vi "ReadWriteLoopCase1.vi"() -> ()   [LabVIEW 2019]
uses:
  <vilib>/DAQmx/read.llb/DAQmx Read (Analog DBL 1Chan 1Samp).vi
  <vilib>/DAQmx/write.llb/DAQmx Write (Analog DBL 1Chan 1Samp).vi
  <vilib>/DAQmx/create/channels.llb/DAQmx Create Channel (AI-Voltage-Basic).vi
  <vilib>/DAQmx/configure/timing.llb/DAQmx Timing (Sample Clock).vi
  <vilib>/DAQmx/create/channels.llb/DAQmx Create Channel (AO-Voltage-Basic).vi
  <vilib>/DAQmx/miscellaneous.llb/DAQmx Fill In Error Info.vi
panel:
  out "error out":errorcluster
  out "Slide":dbl(slide) scale=2900.0..3100.0
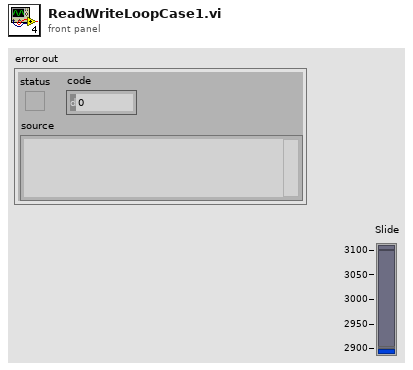
[diagram p1: front panel]
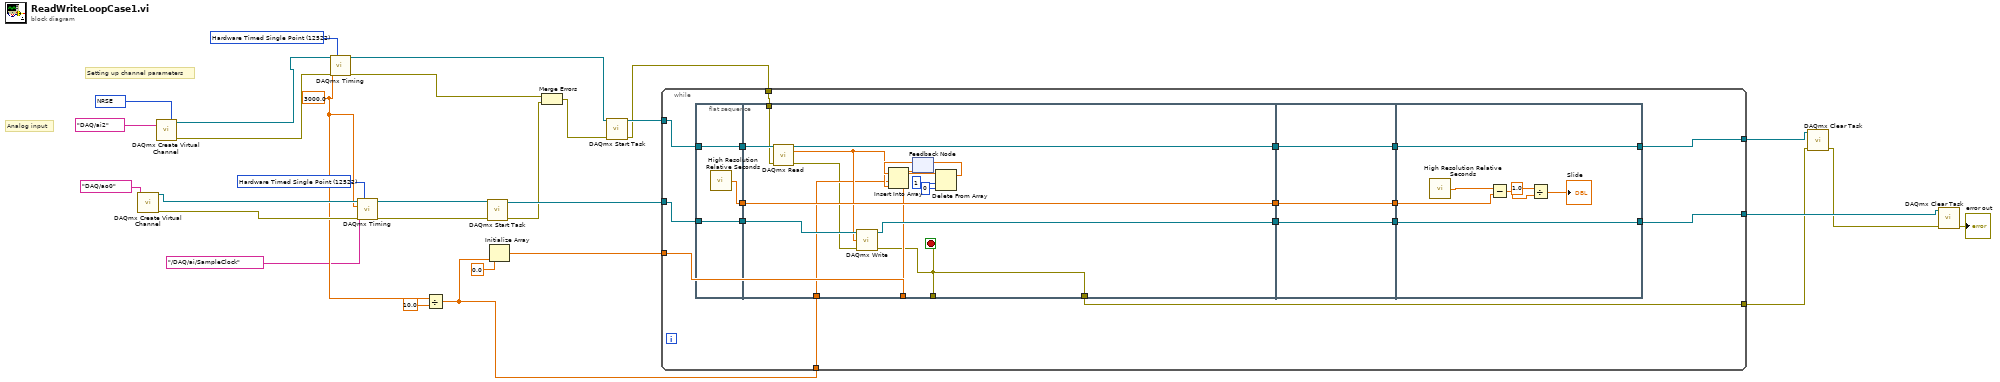
[diagram p0: block diagram]
diagram:
  w3 = 12522 items=["Finite Samples"=10178, "Continuous Samples"=10123, "Hardware Timed Single Point"=12522] ("sample mode")
  w4 = 3000.0 ("rate")
  w24 = 12522 items=["Finite Samples"=10178, "Continuous Samples"=10123, "Hardware Timed Single Point"=12522] ("sample mode")
  w27 = 10078 items=["Default"=-1, "RSE"=10083, "NRSE"=10078, "Differential"=10106, "Pseudodifferential"=12529] ("input terminal configuration")
  # "Analog input"
  # "Setting up channel parameters"
  n1 = call-poly <vilib>:"DAQmx Create Virtual Channel.vi"("physical channels"=tag "DAQ/ao0") -> ("task out"=w8:refnum<k21>, "error out"=w6:errorcluster)  [unwired: 13 in]
  n2 = call-poly <vilib>:"DAQmx Create Virtual Channel.vi"("input terminal configuration"=w27, "physical channels"=tag "DAQ/ai2") -> ("task out"=w25:refnum<k21>, "error out"=w10:errorcluster)  [unwired: 12 in]
  n3 = call-poly <vilib>:"DAQmx Timing.vi"("task/channels in"=w25, "sample mode"=w24, "rate"=w4, "error in"=w10) -> ("task out"=w2:refnum<k21>, "error out"=w9:errorcluster)  [unwired: 10 in]
  n4 = call-poly <vilib>:"DAQmx Timing.vi"("task/channels in"=w8, "sample mode"=w3, "rate"=w4, "source"=tag "/DAQ/ai/SampleClock", "error in"=w6) -> ("task out"=w7:refnum<k21>, "error out"=w5:errorcluster)  [unwired: 9 in]
  n5 = Divide(x=w4, y=10.0) -> (x/y=w19:dbl)
  n6 = call <vilib>:"DAQmx Start Task.vi"("task/channels in"=w7, "error in"=w5) -> ("task out"=w28:refnum<k21>, "error out"=w18:errorcluster)  [unwired: 12 in]
  n7 = Initialize Array(0.0 ("element"), w19) -> (w22:dbl[])
  n8 = Merge Errors(w9, w18) -> (w17:errorcluster)
  n9 = call <vilib>:"DAQmx Start Task.vi"("task/channels in"=w2, "error in"=w17) -> ("task out"=w29:refnum<k21>, "error out"=w16:errorcluster)  [unwired: 12 in]
  n10 = while {
    tunnel: w29 -> [w46]
    tunnel: w28 -> [w45]
    tunnel: [w44] -> w15
    tunnel: [w43] -> w14
    tunnel: w22 -> [w33]
    tunnel: w19 -> [w32]
    tunnel: w16 -> [w31]
    tunnel: [w30] -> w13
    stop <- w47 stop-if-true
    n11 = flat-sequence {
      tunnel: w45 -> [w49]
      tunnel: w46 -> [w50]
      tunnel: [w50] -> w42
      tunnel: [w49] -> w41
      tunnel: [w48] -> w34
      tunnel: [w51] -> w47
      tunnel: w42 -> [w66]
      tunnel: w41 -> [w65]
      tunnel: [w64] -> w40
      tunnel: [w63] -> w39
      tunnel: [w62] -> w35
      tunnel: w34 -> [w62]
      tunnel: w33 -> [w58]
      tunnel: w32 -> [w54]
      tunnel: w31 -> [w53]
      tunnel: [w51] -> w30
      tunnel: w40 -> [w69]
      tunnel: w39 -> [w68]
      tunnel: [w69] -> w38
      tunnel: [w68] -> w37
      tunnel: [w67] -> w36
      tunnel: w35 -> [w67]
      tunnel: [w70] -> w43
      tunnel: [w76] -> w44
      tunnel: w38 -> [w76]
      tunnel: w37 -> [w70]
      tunnel: w36 -> [w74]
      frame #0 {
        n12 = call <vilib>:"High Resolution Relative Seconds.vi"() -> ("relative seconds"=w48:dbl)
      }
      frame #1 {
        n13 = call-poly <vilib>:"DAQmx Read.vi"("task/channels in"=w66, "error in"=w53) -> ("task out"=w64:refnum<k21>, "data"=w55:dbl, "error out"=w52:errorcluster)  [unwired: 11 in]
        n14 = call-poly <vilib>:"DAQmx Write.vi"("task/channels in"=w65, "data"=w55, "error in"=w52) -> ("task out"=w63:refnum<k21>, "error out"=w51:errorcluster)  [unwired: 10 in, 1 out]
        n15 = feedback #1(w58) -> (w61:dbl[])
        n16 = Insert Into Array(array=w61, index=w54, new element=w55) -> (w57:dbl[])
        n17 = Delete From Array(array=w57, length=1, index=0) -> (array with subset deleted=w56:dbl[])  [unwired: 1 out]
        n18 = feedback-in #1(w56) -> ()
      }
      frame #2 {
      }
      frame #3 {
        n19 = call <vilib>:"High Resolution Relative Seconds.vi"() -> ("relative seconds"=w75:dbl)
        n20 = Subtract(x=w75, y=w74) -> (x-y=w72:dbl)
        n21 = Divide(x=1.0, y=w72) -> (x/y=→"Slide":dbl)
      }
    }
  }
  n22 = call <vilib>:"DAQmx Clear Task.vi"("task in"=w15, "error in"=w13) -> ("error out"=w12:errorcluster)  [unwired: 13 in]
  n23 = call <vilib>:"DAQmx Clear Task.vi"("task in"=w14, "error in"=w12) -> ("error out"=→"error out":errorcluster)  [unwired: 13 in]
